vi "Create Channel Cluster.vi"(8 "error in":errorcluster, 10 "Settings Cluster Path":path, 11 "Node":refnum<k20>) -> (0 "error out":errorcluster, 1 "Clust Refnum":refnum<vi>, 2 "Channel Type":string, 3 "Node":refnum<k20>)   [LabVIEW 2026, in "Plugin XML Parser.lvlib"]
uses:
  Plugin XML Parser.lvlib
  <vilib>/numeric/LVNumericRepresentation.ctl
  <vilib>/Utility/miscctls.llb/LVPositionTypeDef.ctl
  <vilib>/xml/Close Reference(Node).vi
  <resource>/objmgr/DOMUserDefRef.rc
  <vilib>/xml/NI_XML.lvlib
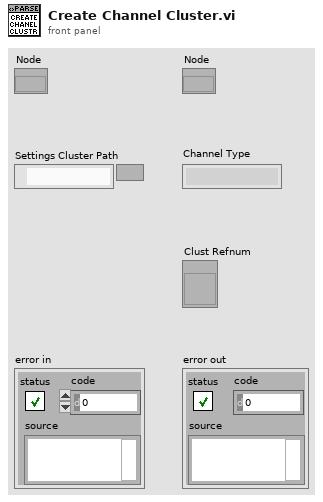
[diagram p1: front panel]
types:
  T1 = typedef "LVNumericRepresentation.ctl" = enum32{"Extended Precision", "Double Precision", "Single Precision", "Long", "Word", "Byte", "Unsigned Long", "Unsigned Word", "Unsigned Byte", "Complex Extended", "Complex Double", "Complex Single", "Quad", "Unsigned Quad", "Fixed-Point"}
  T2 = typedef "LVPositionTypeDef.ctl" = cluster{"Left":i32, "Top":i32}
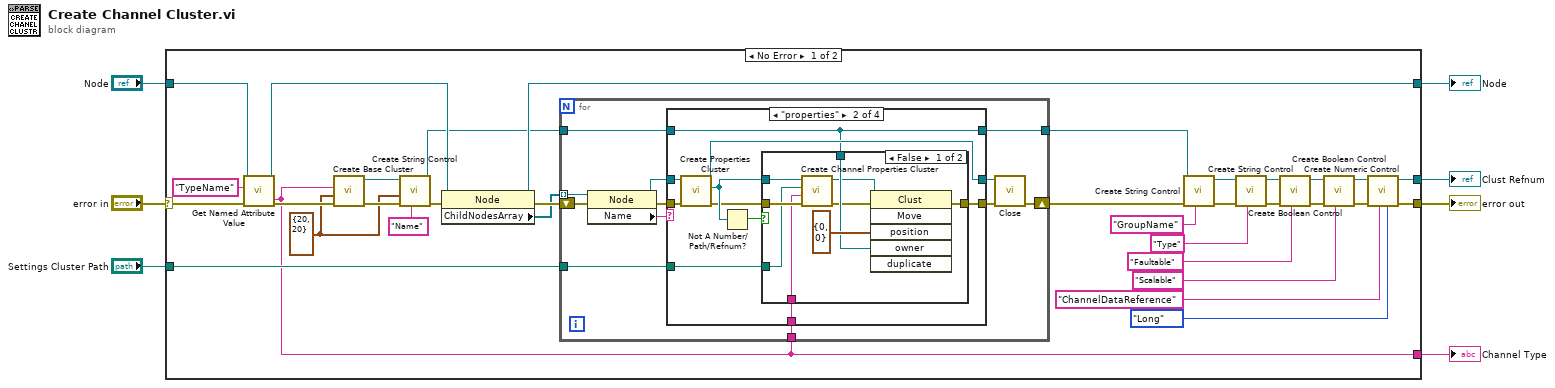
[diagram p0: block diagram]
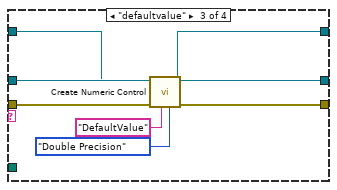
[diagram p4: hidden frame]
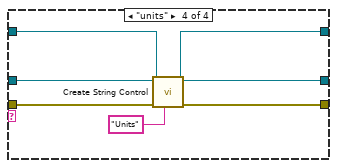
[diagram p5: hidden frame]
diagram:
  n1 = case shown="No Error" "error in" {
    selector: "error in" -> [w41 w91]
    tunnel: [w33 w91] -> w6
    tunnel: "Node" -> [w29 w90]
    tunnel: [w8 _] -> w4
    tunnel: [w27 w90] -> w3
    tunnel: [w16 _] -> w2
    tunnel: "Settings Cluster Path" -> [w9 _]
    frame No Error {
      w25 = cluster{"Horizontal":i16, "Vertical":i16} {"Horizontal"=20, "Vertical"=20} ("Point")
      n2 = call "Get Named Attribute Value.vi"("error in"=w41, "Attribute Name"="TypeName", "Node In"=w29) -> ("error out"=w40:errorcluster, "Node Out"=w28:refnum<k20>, "Attribute Value"=w8:string)  [unwired: 5 in, 1 out]
      n3 = call "Create Base Cluster.vi"("error in"=w40, "Location"=w25, "Cluster Name"=w8) -> ("error out"=w38:errorcluster, "Cluster out"=w24:refnum<vi>)  [unwired: 6 in, 1 out]
      n4 = call "Create String Control.vi"("Label.Text"="Name", "error in"=w38, "location"=w25, "Cluster in"=w24) -> ("error out"=w37:errorcluster, "Cluster out"=w23:refnum<vi>)  [unwired: 6 in]
      n5 = property class="Node"(reference=w28, error in=w37) -> (reference out=w27:refnum<k20>, error out=w39:errorcluster, "ChildNodesArray"=w30:refnum<k20>[])
      n6 = for {
        tunnel: w30 -> [w49] mode=indexing
        shift-right: [w50] -> w32
        shift-left: w39 -> [w53]
        tunnel: w23 -> [w46]
        tunnel: [w45] -> w12
        tunnel: w9 -> [w43]
        tunnel: w8 -> [w42]
        n7 = property class="Node"(reference=w49, error in=w53) -> (reference out=w48:refnum<k20>, error out=w52:errorcluster, "Name"=w44:string)
        n8 = case shown="\"properties\"" w44 {
          tunnel: w48 -> [w55 w64 w81 w84]
          tunnel: [w55 w63 w81 w84] -> w47
          tunnel: w46 -> [w54 w61 w80 w87]
          tunnel: w52 -> [w56 w66 w83 w89]
          tunnel: [w56 w65 w82 w88] -> w51
          tunnel: [w54 w61 w79 w86] -> w45
          tunnel: w43 -> [_ w58 _ _]
          tunnel: w42 -> [_ w57 _ _]
          frame Default {
          }
          frame "properties" {
            n9 = call "Create Properties Cluster.vi"("error in"=w66, "Node In"=w64) -> ("error out"=w59:errorcluster, "Clust Refnum"=w60:refnum<vi>, "Node Out"=w63:refnum<k20>)  [unwired: 7 in]
            n10 = Not A Number/Path/Refnum?(number/path/refnum=w60) -> (NaN/Path/Refnum?=w62:bool)
            n11 = case shown="False" w62 {
              tunnel: w61 -> [w73 _]
              tunnel: w59 -> [w72 w76]
              tunnel: [w75 w76] -> w65
              tunnel: w60 -> [w70 _]
              tunnel: w58 -> [w68 _]
              tunnel: w57 -> [w67 _]
              frame False {
                n12 = call "Create Channel Properties Cluster.vi"("error in"=w72, "Channel Type"=w67, "Settings Cluster Path"=w68, "Clust Refnum"=w70) -> ("error out"=w71:errorcluster, "Clust Refnum"=w69:refnum<vi>)  [unwired: 6 in]
                n13 = invoke class="Clust" method="Move"(reference=w69, error in=w71, "position"=T2 {"Left"=0, "Top"=0}, "owner"=w73) -> (error out=w75:errorcluster)  [unwired: 2 in, 5 out]
              }
              frame True {
              }
            }
          }
          frame "defaultvalue" {
            n14 = call "Create Numeric Control.vi"("Representation"=LVNumericRepresentation."Double Precision", "Label.Text"="DefaultValue", "error in"=w83, "Cluster in"=w80) -> ("error out"=w82:errorcluster, "Cluster out"=w79:refnum<vi>)  [unwired: 6 in]
          }
          frame "units" {
            n15 = call "Create String Control.vi"("Label.Text"="Units", "error in"=w89, "Cluster in"=w87) -> ("error out"=w88:errorcluster, "Cluster out"=w86:refnum<vi>)  [unwired: 7 in]
          }
        }
        n16 = call-poly <vilib>:"Close.vi"("error in (no error)"=w51, "node"=w47) -> ("error out"=w50:errorcluster)  [unwired: 7 in]
      }
      n17 = call "Create String Control.vi"("Label.Text"="GroupName", "error in"=w32, "Cluster in"=w12) -> ("error out"=w31:errorcluster, "Cluster out"=w11:refnum<vi>)  [unwired: 7 in]
      n18 = call "Create String Control.vi"("Label.Text"="Type", "error in"=w31, "Cluster in"=w11) -> ("error out"=w36:errorcluster, "Cluster out"=w21:refnum<vi>)  [unwired: 7 in]
      n19 = call "Create Boolean Control.vi"("Label.Text"="Faultable", "error in"=w36, "Cluster in"=w21) -> ("error out"=w35:errorcluster, "Cluster out"=w19:refnum<vi>)  [unwired: 7 in]
      n20 = call "Create Boolean Control.vi"("Label.Text"="Scalable", "error in"=w35, "Cluster in"=w19) -> ("error out"=w34:errorcluster, "Cluster out"=w17:refnum<vi>)  [unwired: 7 in]
      n21 = call "Create Numeric Control.vi"("Representation"=LVNumericRepresentation."Long", "Label.Text"="ChannelDataReference", "error in"=w34, "Cluster in"=w17) -> ("error out"=w33:errorcluster, "Cluster out"=w16:refnum<vi>)  [unwired: 6 in]
    }
    frame Error {
    }
  }
  "Node" <- w3
  "error out" <- w6
  "Channel Type" <- w4
  "Clust Refnum" <- w2
